vi "Enqueue.vi"(7 "Priority (F)":bool, 8 "error in (no error)":errorcluster, 9 "Message Data":variant, 10 "Message":string, 11 "MessageQueue":refnum<queue>) -> (0 "error out":errorcluster, 3 "MessageQueue":refnum<queue>)   [LabVIEW 2014, in "EventModule.lvlib"]
uses:
  EventModule.lvlib
  PublicAPI/Arguments/Messages/clMessage.ctl
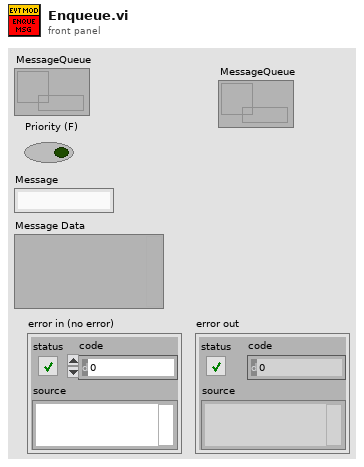
[diagram p1: front panel]
types:
  T1 = typedef "EventModule.lvlib/clMessage.ctl" = cluster{"Message":string, "Message Data":variant}
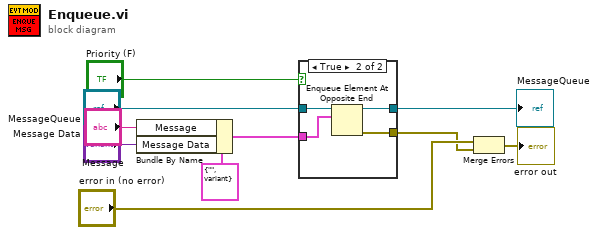
[diagram p0: block diagram]
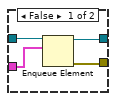
[diagram p2: hidden frame]
diagram:
  n1 = Bundle By Name(cluster=T1 {"Message"="", "Message Data"=variant} ("clMessage"), "Message"="Message", "Message Data"="Message Data") -> (w9:T1)
  n2 = case shown="True" "Priority (F)" {
    tunnel: w9 -> [w13 w18]
    tunnel: "MessageQueue" -> [w14 w17]
    tunnel: [w11 w16] -> w5
    tunnel: [w12 w15] -> w3
    frame False {
      n3 = Enqueue Element(queue=w14, element=w13) -> (queue out=w11:refnum<queue>, error out=w12:errorcluster)  [unwired: 2 in, 1 out]
    }
    frame True {
      n4 = Enqueue Element At Opposite End(queue=w17, element=w18) -> (queue out=w16:refnum<queue>, error out=w15:errorcluster)  [unwired: 2 in, 1 out]
    }
  }
  "MessageQueue" <- w5
  n5 = Merge Errors("error in (no error)", w3) -> (→"error out":errorcluster)
